vi "LJM logger condition register arrays (logger config).vi"(3 "Access?":bool[](array[boolean])=[TRUE, TRUE, TRUE, TRUE, FALSE, FALSE, FALSE, FALSE, FALSE, FALSE, FALSE, FALSE, FALSE, FALSE, FALSE, FALSE], 4 "Values":dbl[](array[numeric])=[2.5, 12345.0] format="%.2f", 5 "Names":string[](array[string])=["DAC0", "TEST_UINT16"]) -> (1 "Values Out":dbl[](array[numeric]), 2 "Names Out":string[](array[string]))   [LabVIEW 2026]
panel:
  # "Trims \"Names\" and \"Values\" arrays according to the boolean \"Access?\" array. Also removes empty register names."
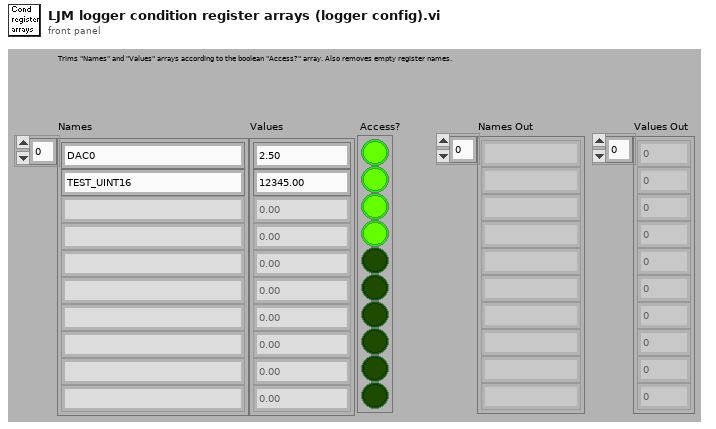
[diagram p1: front panel]
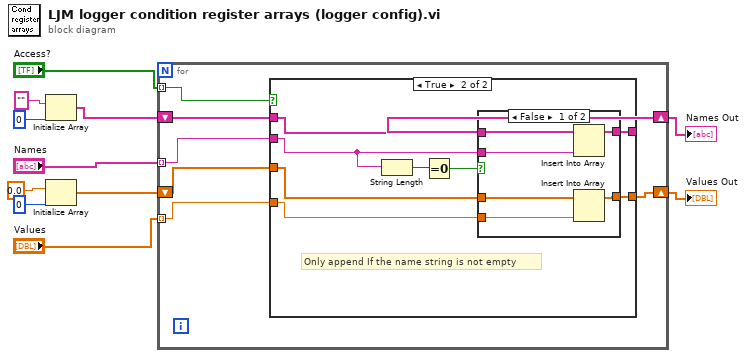
[diagram p0: block diagram]
diagram:
  n1 = Initialize Array("", 0 ("dimension size")) -> (w9:string[])
  n2 = Initialize Array(0.0, 0 ("dimension size")) -> (w3:dbl[])
  n3 = for {
    tunnel: "Names" -> [w17] mode=indexing
    tunnel: "Access?" -> [w15] mode=indexing
    tunnel: "Values" -> [w13] mode=indexing
    shift-right: [w12] -> w1
    shift-left: w3 -> [w14]
    shift-right: [w16] -> w7
    shift-left: w9 -> [w18]
    n4 = case shown="True" w15 {
      tunnel: w18 -> [w20 w28]
      tunnel: w17 -> [_ w21]
      tunnel: [w20 w27] -> w16
      tunnel: w14 -> [w19 w25]
      tunnel: w13 -> [_ w26]
      tunnel: [w19 w24] -> w12
      frame False {
      }
      frame True {
        # "Only append If the name string is not empty"
        n5 = String Length(string=w21) -> (length=w23:i32)
        n6 = Equal To 0?(x=w23) -> (x = 0?=w22:bool)
        n7 = case shown="False" w22 {
          tunnel: w28 -> [w34 w36]
          tunnel: w21 -> [w33 _]
          tunnel: [w32 w36] -> w27
          tunnel: w26 -> [w31 _]
          tunnel: w25 -> [w30 w35]
          tunnel: [w29 w35] -> w24
          frame False {
            n8 = Insert Into Array(array=w34, new element=w33) -> (w32:string[])  [unwired: 1 in]
            n9 = Insert Into Array(array=w30, new element=w31) -> (w29:dbl[])  [unwired: 1 in]
          }
          frame True {
          }
        }
      }
    }
  }
  "Names Out" <- w7
  "Values Out" <- w1
